vi "Step response.vi"() -> ()   [LabVIEW 2014]
panel:
  out "XY Graph 2":cluster{dbl[], "Data":dbl[]}(graph)
  out "XY Graph":cluster{dbl[], "Data":dbl[]}[](graph)
  out "Data rate (Hz)":dbl=20000.0
  out "Real position (um)":dbl[](array[numeric])
  out "Target position (um)":dbl[](array[numeric])
  in  "Step size (um)":dbl caption="Numeric" format="%.6f"
  in  "axis":u32
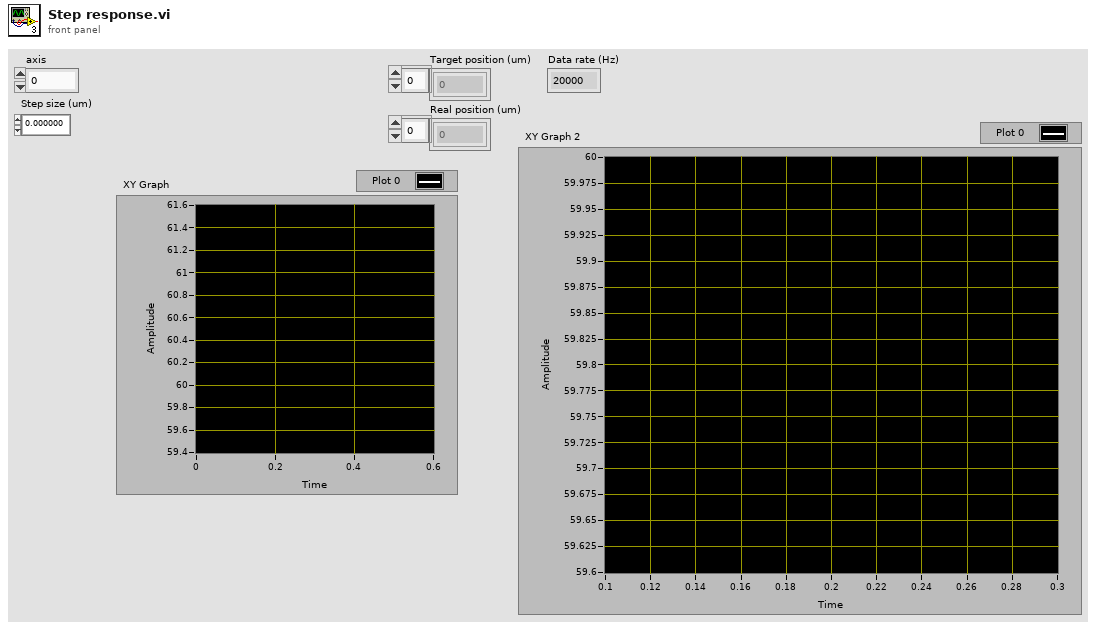
[diagram p1: front panel]
types:
  T1 = enum16{"Target position", "Current position", "position error"}
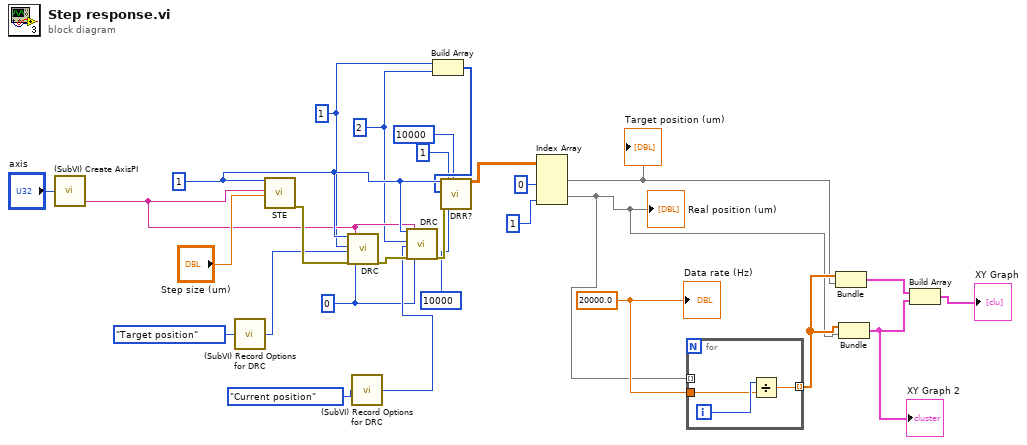
[diagram p0: block diagram]
diagram:
  w9 = 20000.0
  w17 = 0 ("Trigger option")
  w15 = 2 ("Rec. table")
  w16 = 1 ("Rec. table")
  w20 = 1 ("System no.")
  n1 = call "(SubVI) Create AxisPI.vi"("axis"="axis") -> ("Axis String"=w19:string)  [unwired: 2 in, 2 out]
  n2 = call "(SubVI) Record Options for DRC.vi"("Enum"=T1."Target position") -> ("Record options"=w25:i32)  [unwired: 4 in]
  n3 = call "STE.vi"("System no."=w20, "Axis to command"=w19, "Step size"="Step size (um)") -> ("error out"=w26:errorcluster)  [unwired: 3 in, 13 out]
  n4 = call "DRC.vi"("System no."=w20, "Rec. table"=w16, "Rec. option"=w25, "error in"=w26, "Source ID"=w19, "Trigger option"=w17) -> ("error out"=w23:errorcluster)  [unwired: 13 out]
  n5 = call "(SubVI) Record Options for DRC.vi"("Enum"=T1."Current position") -> ("Record options"=w21:i32)  [unwired: 4 in]
  n6 = call "DRC.vi"("System no."=w20, "Rec. table"=w15, "Rec. option"=w21, "error in"=w23, "Source ID"=w19, "Trigger option"=w17) -> ("error out"=w18:errorcluster)  [unwired: 13 out]
  n7 = Build Array(w16, w15) -> (w14:i32[])
  n8 = call "DRR?.vi"("System no."=w20, "Rec. table IDs"=w14, "error in"=w18, "Xo"=1, "N"=10000, "Nmax"=10000) -> ("Data"=w12:dbl[][])  [unwired: 2 in, 11 out]
  n9 = Index Array(array=w12, index (col) #1=0 ("disabled index (col)"), index (col) #2=1 ("disabled index (col)")) -> (element #1=w7:dbl[], element #2=w6:dbl[])  [unwired: 2 in]
  "Target position (um)" <- w7
  "Real position (um)" <- w6
  n10 = for {
    tunnel: w6 -> [_] mode=indexing
    tunnel: w9 -> [w30]
    tunnel: [w29] -> w8 mode=indexing
    i -> [w31]
    n11 = Divide(x=w31, y=w30) -> (x/y=w29:dbl)
  }
  n12 = Bundle(w8, "Data"=w7) -> (w5:cluster{dbl[], "Data":dbl[]})  [unwired: 1 in]
  n13 = Bundle(w8, "Data"=w6) -> (w1:cluster{dbl[], "Data":dbl[]})  [unwired: 1 in]
  "XY Graph 2" <- w1
  n14 = Build Array(w5, w1) -> (→"XY Graph":cluster{dbl[], "Data":dbl[]}[])
  "Data rate (Hz)" <- w9
